vi "PopulateTargetRing.vi"(8 "error in (no error)":errorcluster, 10 "ring info":refnum<class "RingItem.lvclass">[](array[class]), 11 "Targets ring":refnum<vi>) -> (0 "error out":errorcluster, 2 "ring info out":refnum<class "RingItem.lvclass">[](array[class]))   [LabVIEW 2009, in "NavScreen.lvlib"]
uses:
  NavScreen.lvlib
  Classes/RingItem/RingItem.lvclass
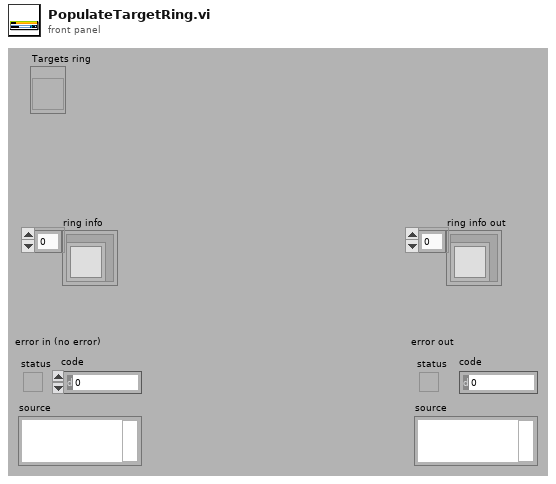
[diagram p1: front panel]
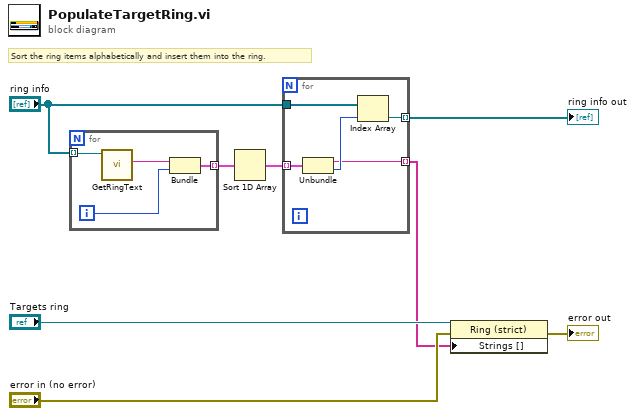
[diagram p0: block diagram]
diagram:
  # "Sort the ring items alphabetically and insert them into the ring."
  n1 = for {
    tunnel: "ring info" -> [w12] mode=indexing
    tunnel: [w9] -> w5 mode=indexing
    i -> [w10]
    n2 = call "GetRingText.vi"("RingItem in"=w12) -> ("ring text"=w11:string)  [unwired: 8 in, 2 out]
    n3 = Bundle("ring text"=w11, w10) -> (w9:cluster{"ring text":string, i32})  [unwired: 1 in]
  }
  n4 = Sort 1D Array(array=w5) -> (sorted array=w4:cluster{"ring text":string, i32}[])
  n5 = for {
    tunnel: w4 -> [w16] mode=indexing
    tunnel: "ring info" -> [w17]
    tunnel: [w14] -> w1 mode=indexing
    tunnel: [w13] -> w2 mode=indexing
    n6 = Unbundle(w16) -> ("ring text"=w14:string, w15:i32)
    n7 = Index Array(array=w17, index=w15) -> (element=w13:refnum<class "RingItem.lvclass">)
  }
  "ring info out" <- w2
  n8 = property on="Property Node" class="Ring (strict)"(reference="Targets ring", error in="error in (no error)", "Strings []"=w1) -> (error out=→"error out":errorcluster)  [unwired: 1 out]
